vi "Autonomous Indictacotr.vi"() -> ()   [LabVIEW 2014]
panel:
  out "String Out":string
  in  "Int In":dbl
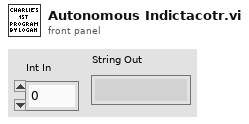
[diagram p1: front panel]
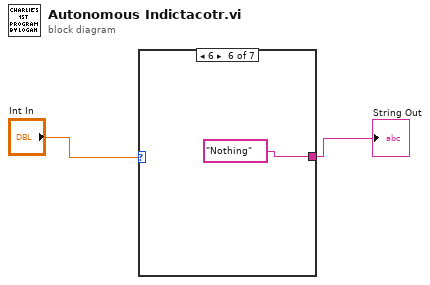
[diagram p0: block diagram]
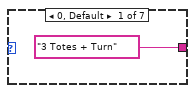
[diagram p2: hidden frame]
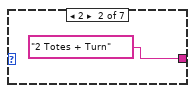
[diagram p3: hidden frame]
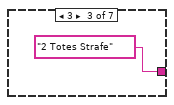
[diagram p4: hidden frame]
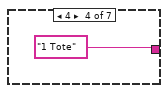
[diagram p5: hidden frame]
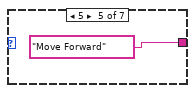
[diagram p6: hidden frame]
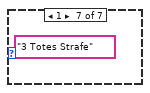
[diagram p7: hidden frame]
diagram:
  n1 = case shown="6" "Int In" {
    tunnel: ["3 Totes + Turn" "2 Totes + Turn" "2 Totes Strafe" "1 Tote" "Move Forward" "Nothing" _] -> w1
    frame 0, Default {
    }
    frame 2 {
    }
    frame 3 {
    }
    frame 4 {
    }
    frame 5 {
    }
    frame 6 {
    }
    frame 1 {
      (unwired) "3 Totes Strafe"
    }
  }
  "String Out" <- w1
